vi "C3 to End Switch.vi"(8 "Command Info In":T1, 10 "Block Inputs":T5, 11 "Starting Position":T4) -> (0 "Command Info Out":T1)   [LabVIEW 2017]
uses:
  Block Clusters/C3 to End Switch 2.ctl
  Support Code/Starting Position.ctl
  <vilib>/Rock Robotics/WPI/Framework/Command Status Info.ctl
  <vilib>/Rock Robotics/WPI/Framework/Completion Status.ctl
  <vilib>/Rock Robotics/WPI/Framework/Completion Notifier.ctl
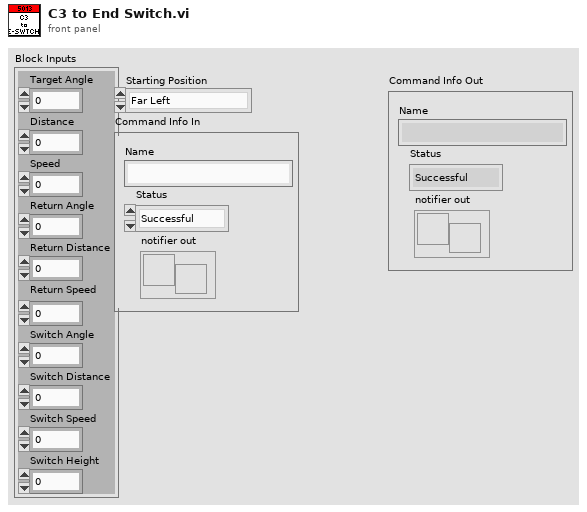
[diagram p1: front panel]
types:
  T1 = typedef "Command Status Info.ctl" = cluster{"Name":string, "Status":T2, "notifier out":T3}
  T2 = typedef "Completion Status.ctl" = enum16{"Successful", "Aborted", "Incomplete"}
  T3 = typedef "Completion Notifier.ctl" = refnum<notifier>
  T4 = typedef "Starting Position.ctl" = enum16{"Far Left", "Center", "Far Right"}
  T5 = typedef "C3 to End Switch 2.ctl" = cluster{"Target Angle":dbl, "Distance":dbl, "Speed":dbl, "Return Angle":dbl, "Return Distance":dbl, "Return Speed":dbl, "Switch Angle":dbl, "Switch Distance":dbl, "Switch Speed":dbl, "Switch Height":dbl}
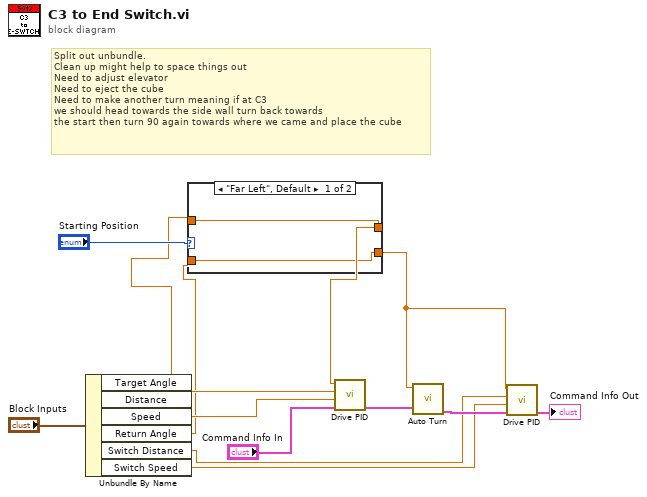
[diagram p0: block diagram]
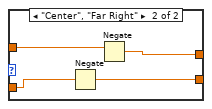
[diagram p2: hidden frame]
diagram:
  # "Split out unbundle.\nClean up might help to space things out\nNeed to adjust elevator\nNeed to eject the cube\nNeed to make another turn meaning if at C3 \nwe should head towards the side wall turn back towards\nthe start then turn 90 again towards where we came and place the cube"
  n1 = Unbundle By Name("Block Inputs") -> ("Target Angle"=w12:dbl, "Distance"=w11:dbl, "Speed"=w10:dbl, "Return Angle"=w5:dbl, "Switch Distance"=w6:dbl, "Switch Speed"=w2:dbl)
  n2 = case shown="\"Far Left\", Default" "Starting Position" {
    tunnel: w12 -> [w16 w20]
    tunnel: [w16 w19] -> w4
    tunnel: w5 -> [w15 w18]
    tunnel: [w15 w17] -> w3
    frame "Far Left", Default {
    }
    frame "Center", "Far Right" {
      n3 = Negate(x=w18) -> (-x=w17:dbl)
      n4 = Negate(x=w20) -> (-x=w19:dbl)
    }
  }
  n5 = call "Drive PID.vi"("Command Info In"="Command Info In", "Speed"=w10, "Distance"=w11, "Target Angle"=w4) -> ("Command Info Out"=w8:T1)  [unwired: 7 in]
  n6 = call "Auto Turn.vi"("Command Info In"=w8, "Target Angle"=w3) -> ("Command Info Out"=w7:T1)  [unwired: 9 in]
  n7 = call "Drive PID.vi"("Command Info In"=w7, "Speed"=w2, "Distance"=w6, "Target Angle"=w3) -> ("Command Info Out"=→"Command Info Out":T1)  [unwired: 7 in]
